vi "Arduino RGB LED I2C.vi"() -> ()   [LabVIEW 2012]
doc: "An example that uses the Arduino's PWM pins to control an RGB LED."
uses:
  <vilib>/LabVIEW Interface for Arduino/LabVIEW Interface for Arduino.lvlib
panel:
  in  "PCA Address":u8(ring)=45 items=["0x2D"=45, "0x2E"=46]
  out "Color":u32(colorbox)
  in  "Blue":u8(slide) scale=0.0..255.0
  in  "Green":u8(slide) scale=0.0..255.0
  in  "Stop":bool
  in  "Red":u8(slide) scale=0.0..255.0
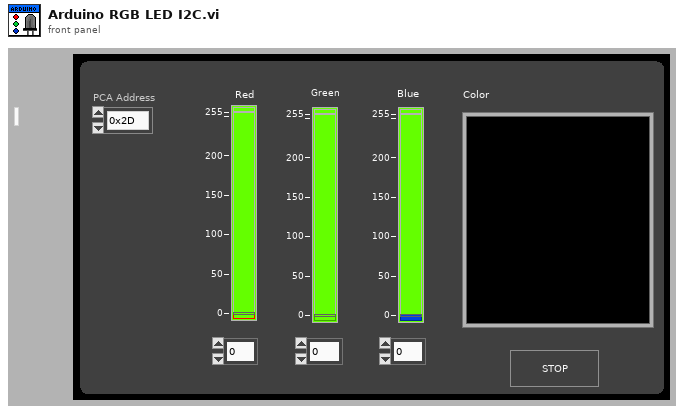
[diagram p1: front panel]
types:
  T1 = typedef "LabVIEW Interface for Arduino.lvlib/Arduino Resource.ctl" = cluster{"VISA resource":refnum<visa-resource-name>, "Board Type":T2, "Connection Type":enum8{"USB / Serial"}, "Bytes Per Packet (15)":u8}
  T2 = typedef "LabVIEW Interface for Arduino.lvlib/Board Type.ctl" = enum16{"Uno", "Dimuelanove w/Atmega 328", "Mega 2560"}
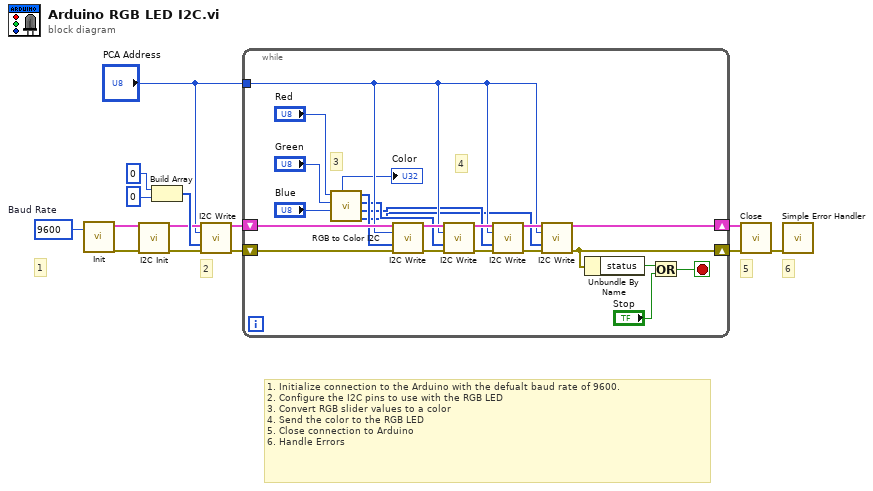
[diagram p0: block diagram]
diagram:
  w4 = u32 9600  # Baud Rate
  # "6"
  # "5"
  # "2"
  # "1"
  # "1. Initialize connection to the Arduino with the defualt baud rate of 9600.\n2. Configure the I2C pins to use with the RGB LED\n3. Convert RGB slider values to a color\n4. Send the color to the RGB LED\n5. Close connection to Arduino\n6. Handle Errors"
  n1 = call <vilib>:"Init.vi"("Baud Rate (115200)"=w4) -> ("Arduino Resource"=w11:T1, "error out"=w10:errorcluster)  [unwired: 17 in]
  n2 = call <vilib>:"I2C Init.vi"("Arduino Resource"=w11, "error in"=w10) -> ("Arduino Resource"=w6:T1, "error out"=w5:errorcluster)  [unwired: 12 in]
  n3 = Build Array(0, 0) -> (w9:i32[])
  n4 = call <vilib>:"I2C Write.vi"("Arduino Resource"=w6, "Address (0)"="PCA Address", "I2C Data Bytes"=w9, "error in"=w5) -> ("Arduino Resource"=w2:T1, "error out"=w1:errorcluster)  [unwired: 10 in]
  n5 = while {
    shift-right: [w28] -> w12
    shift-left: w2 -> [w36]
    shift-right: [w16] -> w14
    shift-left: w1 -> [w35]
    tunnel: "PCA Address" -> [w27]
    stop <- w18 stop-if-true
    # "4"
    # "3"
    n6 = call "RGB to Color I2C.vi"("B"="Blue", "G"="Green", "R"="Red") -> ("LEDout"=w20:i32[], "Blue Color"=w21:i32[], "Green Color"=w22:i32[], "Red Color"=w23:i32[], "Color"=→"Color":u32)  [unwired: 1 in]
    n7 = call <vilib>:"I2C Write.vi"("Arduino Resource"=w36, "Address (0)"=w27, "I2C Data Bytes"=w23, "error in"=w35) -> ("Arduino Resource"=w34:T1, "error out"=w33:errorcluster)  [unwired: 10 in]
    n8 = call <vilib>:"I2C Write.vi"("Arduino Resource"=w34, "Address (0)"=w27, "I2C Data Bytes"=w22, "error in"=w33) -> ("Arduino Resource"=w32:T1, "error out"=w31:errorcluster)  [unwired: 10 in]
    n9 = call <vilib>:"I2C Write.vi"("Arduino Resource"=w32, "Address (0)"=w27, "I2C Data Bytes"=w21, "error in"=w31) -> ("Arduino Resource"=w30:T1, "error out"=w29:errorcluster)  [unwired: 10 in]
    n10 = call <vilib>:"I2C Write.vi"("Arduino Resource"=w30, "Address (0)"=w27, "I2C Data Bytes"=w20, "error in"=w29) -> ("Arduino Resource"=w28:T1, "error out"=w16:errorcluster)  [unwired: 10 in]
    n11 = Unbundle By Name(w16) -> ("status"=w15:bool)
    n12 = Or(x=w15, y="Stop") -> (x .or. y?=w18:bool)
  }
  n13 = call <vilib>:"Close.vi"("Arduino Resource"=w12, "error in"=w14) -> ("error out"=w13:errorcluster)  [unwired: 13 in]
  n14 = call <vilib>:"Simple Error Handler.vi"("error in (no error)"=w13) -> ()  [unwired: 4 in, 5 out]
